vi "Test Helper Loop Broadcast Started State.vi"(8 "error in (no error)":errorcluster, 11 "Helper Loop Test In":refnum<class "Helper Loop Test.lvclass">) -> (0 "error out":errorcluster, 3 "Helper Loop Test Out":refnum<class "Helper Loop Test.lvclass">)   [LabVIEW 2020, in "Helper Loop Test.lvclass"]
uses:
  Helper Loop Test.lvclass
  C:/Program Files (x86)/National Instruments/LabVIEW 2020/vi.lib/Asteme/LUnit/Test Case.lvclass
  Mock Process/Mock Process.lvclass
  C:/Users/anton/Documents/GitHub/Triarc-Framework/source/Framework/Process/Process.lvclass
  Framework/Process/Process.lvclass/Process.ctl
  <vilib>/Asteme/LUnit/Test Case.lvclass/Test Case.ctl
  <vilib>/Asteme/LUnit/LUnit Assertion Result.lvclass/LUnit Assertion Result.ctl
  Framework/Broadcast Event Helpers/Execution timer.vi
  Framework/Process/Private/SubVIs/Wait for finish.vi
  Framework/Process/Protected/Messaging/Enqueue Message.vi
  Framework/Process/Private/SubVIs/Set Lifecycle State.vi
  Framework/Process/Public/Lifecycle/Get Lifecycle State.vi
  <vilib>/Asteme/LUnit/Palette/Pass.vi
  <vilib>/Asteme/LUnit/Palette/Fail.vi
  <vilib>/Asteme/LUnit/Variant to string.vi
  <vilib>/Asteme/LUnit/Set Assertion Type.vi
  <vilib>/Utility/error.llb/Clear Errors.vi
  <vilib>/Asteme/LUnit/Add test result.vi
  <vilib>/Asteme/LUnit/LUnit Write Passed.vi
  <vilib>/Asteme/LUnit/LUnit Get Test Case.vi
  <vilib>/Asteme/LUnit/Assertion Result/LUnit Get Test Name.vi
  <vilib>/Asteme/LUnit/LUnit Write Message.vi
  <vilib>/Asteme/LUnit/LUnit Write Description.vi
  <vilib>/Asteme/LUnit/LUnit Write Assertion Type.vi
  <vilib>/Asteme/LUnit/Read Test Case Name.vi
  Framework/Broadcast Event Helpers/Dequeue Broadcast Message.vi
  <vilib>/Utility/error.llb/Error Cluster From Error Code.vi
  <vilib>/Utility/Data Type/Get Type Information.vi
  <vilib>/Utility/LVClass/Get LV Class Name.vi
  <vilib>/Asteme/LUnit/LUnit Assertion Result.lvclass
  Framework/Process/Process.lvclass
  <vilib>/Asteme/LUnit/Test Case.lvclass
  Framework/Broadcast Event Helpers/Broadcast Event Helpers.lvlib
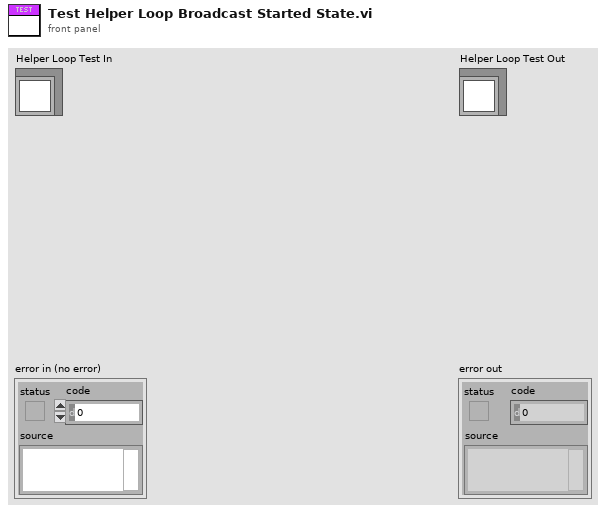
[diagram p1: front panel]
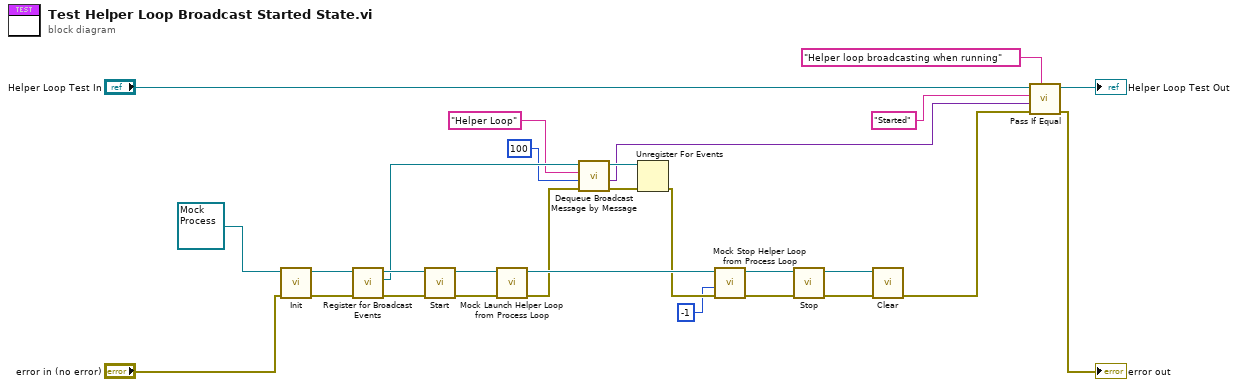
[diagram p0: block diagram]
diagram:
  n1 = call-dynamic "Init.vi"("error in (no error)"="error in (no error)", "Mock Process In"=refnum<class "Mock Process.lvclass"> refnum) -> ("error out"=w26:errorcluster, "Mock Process Out"=w27:refnum<class "Mock Process.lvclass">)  [unwired: 8 in]
  n2 = call "Register for Broadcast Events.vi"("error in (no error)"=w26, "Process In"=w27) -> ("error out"=w24:errorcluster, "Event Registration Refnum Out"=w11:refnum<event-registration>, "Process Out"=w25:refnum<class "Mock Process.lvclass">)  [unwired: 7 in]
  n3 = call "Start.vi"("error in (no error)"=w24, "Process In"=w25) -> ("error out"=w22:errorcluster, "Process Out"=w23:refnum<class "Mock Process.lvclass">)  [unwired: 7 in, 1 out]
  n4 = call "Mock Launch Helper Loop from Process Loop.vi"("error in (no error)"=w22, "Mock Process in"=w23) -> ("error out"=w9:errorcluster, "Mock Process out"=w21:refnum<class "Mock Process.lvclass">)  [unwired: 8 in]
  n5 = call "Dequeue Broadcast Message by Message.vi"("error in (no error)"=w9, "Timeout (-1)"=100, "Message"="Helper Loop" ("y"), "Event Registration Refnum"=w11) -> ("error out"=w3:errorcluster, "Message Data"=w2:variant, "Event Registration Refnum Out"=w8:refnum<event-registration>)  [unwired: 3 in, 2 out]
  n6 = Unregister For Events(event registration refnum=w8, error in=w3) -> (error out=w7:errorcluster)
  n7 = call "Mock Stop Helper Loop from Process Loop.vi"("error in (no error)"=w7, "timeout in ms (-1)"=-1, "Mock Process in"=w21) -> ("error out"=w19:errorcluster, "Mock Process out"=w20:refnum<class "Mock Process.lvclass">)  [unwired: 6 in, 1 out]
  n8 = call "Stop.vi"("error in (no error)"=w19, "Process In"=w20) -> ("error out"=w18:errorcluster, "Process Out"=w1:refnum<class "Mock Process.lvclass">)  [unwired: 7 in, 1 out]
  n9 = call-dynamic "Clear.vi"("error in (no error)"=w18, "Mock Process In"=w1) -> ("error out"=w17:errorcluster)  [unwired: 9 in]
  n10 = call <vilib>:"Pass If Equal.vi"("Description"="Helper loop broadcasting when running", "error in (no error)"=w17, "Actual"=w2, "Expected"="Started" ("Description"), "Test Case In"="Helper Loop Test In") -> ("error out"=→"error out":errorcluster, "Test Case Out"=→"Helper Loop Test Out":refnum<class "Helper Loop Test.lvclass">)  [unwired: 5 in]
